vi "UTILTIY Remove Blank Rows.vi"(10 "all rows in":string[](array[string]), 11 "Numeric":i32) -> (3 "all rows out":string[](array[string]))   [LabVIEW 2018]
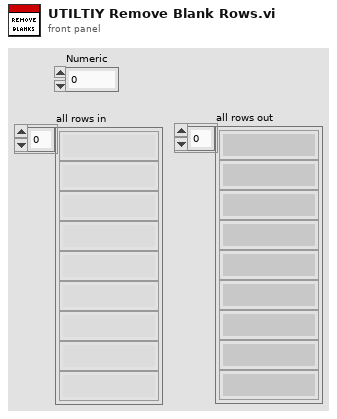
[diagram p1: front panel]
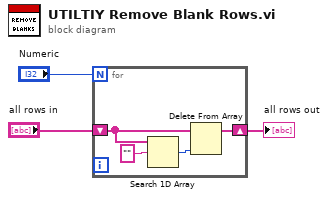
[diagram p0: block diagram]
diagram:
  n1 = for {
    N: "Numeric" -> [_]
    shift-right: [w4] -> w3
    shift-left: "all rows in" -> [w6]
    n2 = Search 1D Array(1D array=w6, element="") -> (index of element=w5:i32)  [unwired: 1 in]
    n3 = Delete From Array(array=w6, index=w5) -> (array with subset deleted=w4:string[])  [unwired: 1 in, 1 out]
  }
  "all rows out" <- w3
